vi "Merge Table Data.vi"(8 "error in (no error)":errorcluster, 9 "Merge Default Values? (F)":bool, 10 "Table to Merge":refnum<class "Basic Table.lvclass">, 11 "Basic Table in":refnum<class "Basic Table.lvclass">) -> (0 "error out":errorcluster, 3 "Basic Table out":refnum<class "Basic Table.lvclass">)   [LabVIEW 2020, in "Table.lvlib" / "Basic Table.lvclass"]
uses:
  Basic Table.lvclass
  Column Libraries/Column Interface/Column Interface Class/Column Interface.lvclass
  Basic Table.lvclass/Basic Table.ctl
  Table Configuration Interface/Table Configuration Interface.lvclass
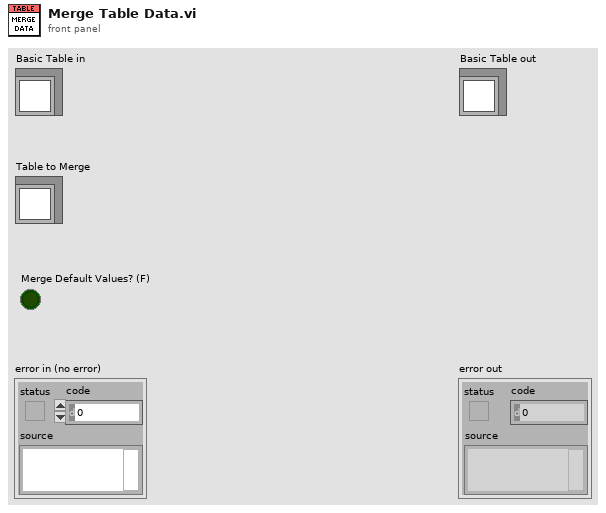
[diagram p1: front panel]
types:
  T1 = map{string, refnum<class "Column Interface.lvclass">}
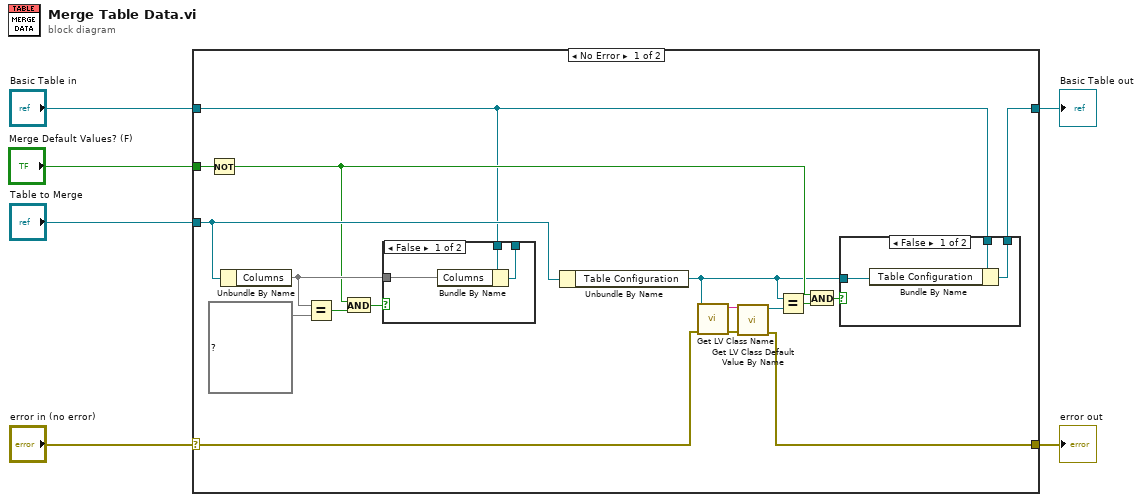
[diagram p0: block diagram]
diagram:
  n1 = case shown="No Error" "error in (no error)" {
    selector: "error in (no error)" -> [w8 w33]
    tunnel: [w7 w33] -> w5
    tunnel: [w10 w32] -> w3
    tunnel: "Basic Table in" -> [w11 w32]
    tunnel: "Table to Merge" -> [w18 _]
    tunnel: "Merge Default Values? (F)" -> [w22 _]
    frame No Error {
      n2 = Not(x=w22) -> (.not. x?=w12:bool)
      n3 = Unbundle By Name(w18) -> ("Columns"=w19:T1)
      n4 = Equal?(x=w19, y=T1 {} ("Columns")) -> (x = y?=w20:bool)
      n5 = And(x=w12, y=w20) -> (x .and. y?=w21:bool)
      n6 = case shown="False" w21 {
        tunnel: w11 -> [w30 w31]
        tunnel: [w29 w31] -> _
        tunnel: w19 -> [w28 _]
        frame False {
          n7 = Bundle By Name(cluster=w30, "Columns"=w28) -> (w29:refnum<class "Basic Table.lvclass">)
        }
        frame True {
        }
      }
      n8 = Unbundle By Name(w18) -> ("Table Configuration"=w9:refnum<class "Table Configuration Interface.lvclass">)
      n9 = call <vilib>:"Get LV Class Name.vi"("error in (no error)"=w8, "object"=w9) -> ("error out"=w17:errorcluster, "class name"=w16:string)  [unwired: 8 in]
      n10 = call <vilib>:"Get LV Class Default Value By Name.vi"("error in (no error)"=w17, "class name"=w16) -> ("error out"=w7:errorcluster, "object"=w15:refnum<class>)  [unwired: 8 in]
      n11 = Equal?(x=w9, y=w15) -> (x = y?=w14:bool)
      n12 = And(x=w12, y=w14) -> (x .and. y?=w13:bool)
      n13 = case shown="False" w13 {
        tunnel: w11 -> [w26 w27]
        tunnel: [w25 w27] -> w10
        tunnel: w9 -> [w24 _]
        frame False {
          n14 = Bundle By Name(cluster=w26, "Table Configuration"=w24) -> (w25:refnum<class "Basic Table.lvclass">)
        }
        frame True {
        }
      }
    }
    frame Error {
    }
  }
  "error out" <- w5
  "Basic Table out" <- w3
